vi "EMG.vi"(8 "error in (no error)":errorcluster caption="错误输入（无错误）", 10 "EMG In":bool, 11 "Step":enum16{"Initial", "Write", "Read"}(ring)) -> (0 "error out":errorcluster caption="错误输出", 3 "EMG Out":bool)   [LabVIEW 2017]
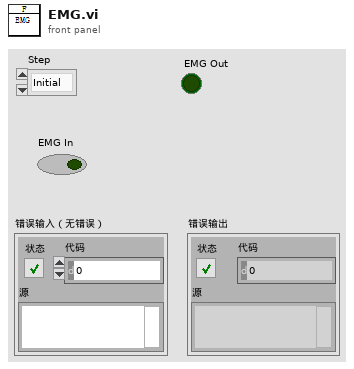
[diagram p1: front panel]
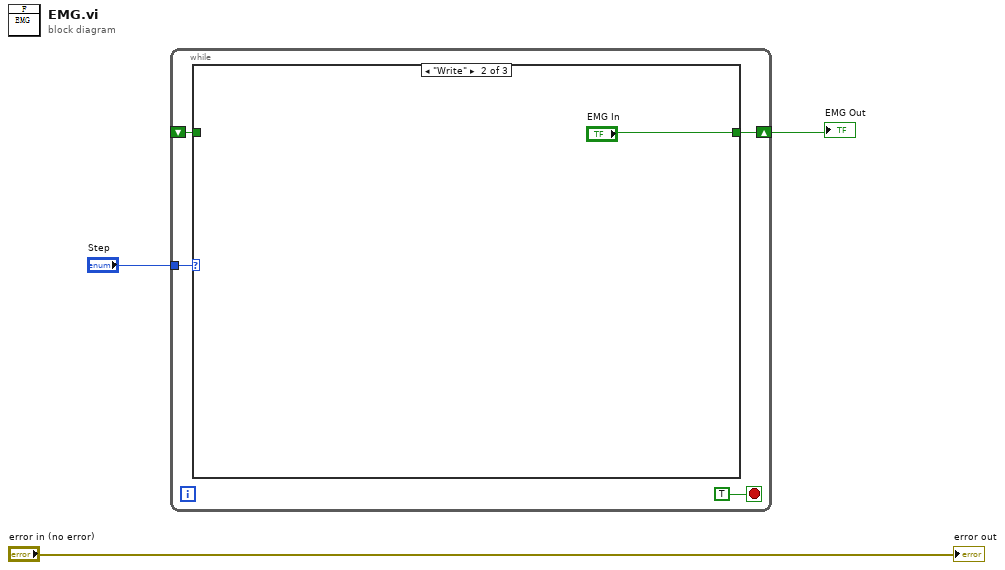
[diagram p0: block diagram]
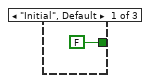
[diagram p2: hidden frame]
diagram:
  n1 = while {
    tunnel: "Step" -> [w7]
    shift-right: [w6] -> w1
    shift-left: _ -> [w4]
    stop <- TRUE stop-if-true
    n2 = case shown="\"Write\"" w7 {
      tunnel: [FALSE "EMG In" w10] -> w6
      tunnel: w4 -> [_ _ w10]
      frame "Initial", Default {
      }
      frame "Write" {
      }
      frame "Read" {
      }
    }
  }
  "EMG Out" <- w1
  "error out" <- "error in (no error)"
